vi "运维调试_总磷总氮.vi"() -> ()   [LabVIEW 2016, in "斯坦道通用流路CODmn.lvlib"]
uses:
  <vilib>/Utility/miscctls.llb/LVPointTypeDef.ctl
  <vilib>/Plasmionique/MB Master/MB_Master/MB_Master.lvclass
  <vilib>/ptbypt/NI_PtbyPt.lvlib
panel:
  out "步骤":u16
  out "seconds since 1Jan1904 2":timestamp
  out "seconds since 1Jan1904":timestamp
  in  "周期设置":bool
  in  "流程操作":bool
  out "消解压力":sgl format="%#.2f kPa"
  out "权限等级":string
  out "总步数":i32
  out "滑动杆":dbl(slide) caption="测试进度" scale=0.0..100.0
  out "试剂余量显示":sgl[][](graph)
  in  "仪器校准":bool
  in  "参数查询":bool
  out "简易步骤名称":string
  in  "温度曲线":bool
  in  "试剂余量":bool
  in  "灯值调整":bool
  out "固件版本号":string
  out "模块版本号":string
  out "注射器温度":sgl format="%#.2f ℃"
  out "消解温度":sgl format="%#.2f ℃"
  out "ADC":sgl
  out "F3":sgl format="%#.6f"
  out "F2":sgl format="%#.6f"
  out "F1":sgl format="%#.6f"
  out "F0":sgl format="%#.6f"
  out "运行状态":T1 {"数据时间:" format="%<%y/%m/%d %H:%M:%S>T"; "仪器时间:" format="%<%y/%m/%d %H:%M:%S>T"}
  in  "单选按钮":T2=enum."总氮"
  in  "布尔":bool
  in  "外设固件":bool
  out "字符串 2":string
  in  "数组":string[](array[string])
  in  "返回":bool
  in  "参数设置":bool
  out "集成报警信息":string
  in  "停止":bool
  in  "手动启动":bool
  in  "调试":bool
  out "多列列表框":i32(listbox)
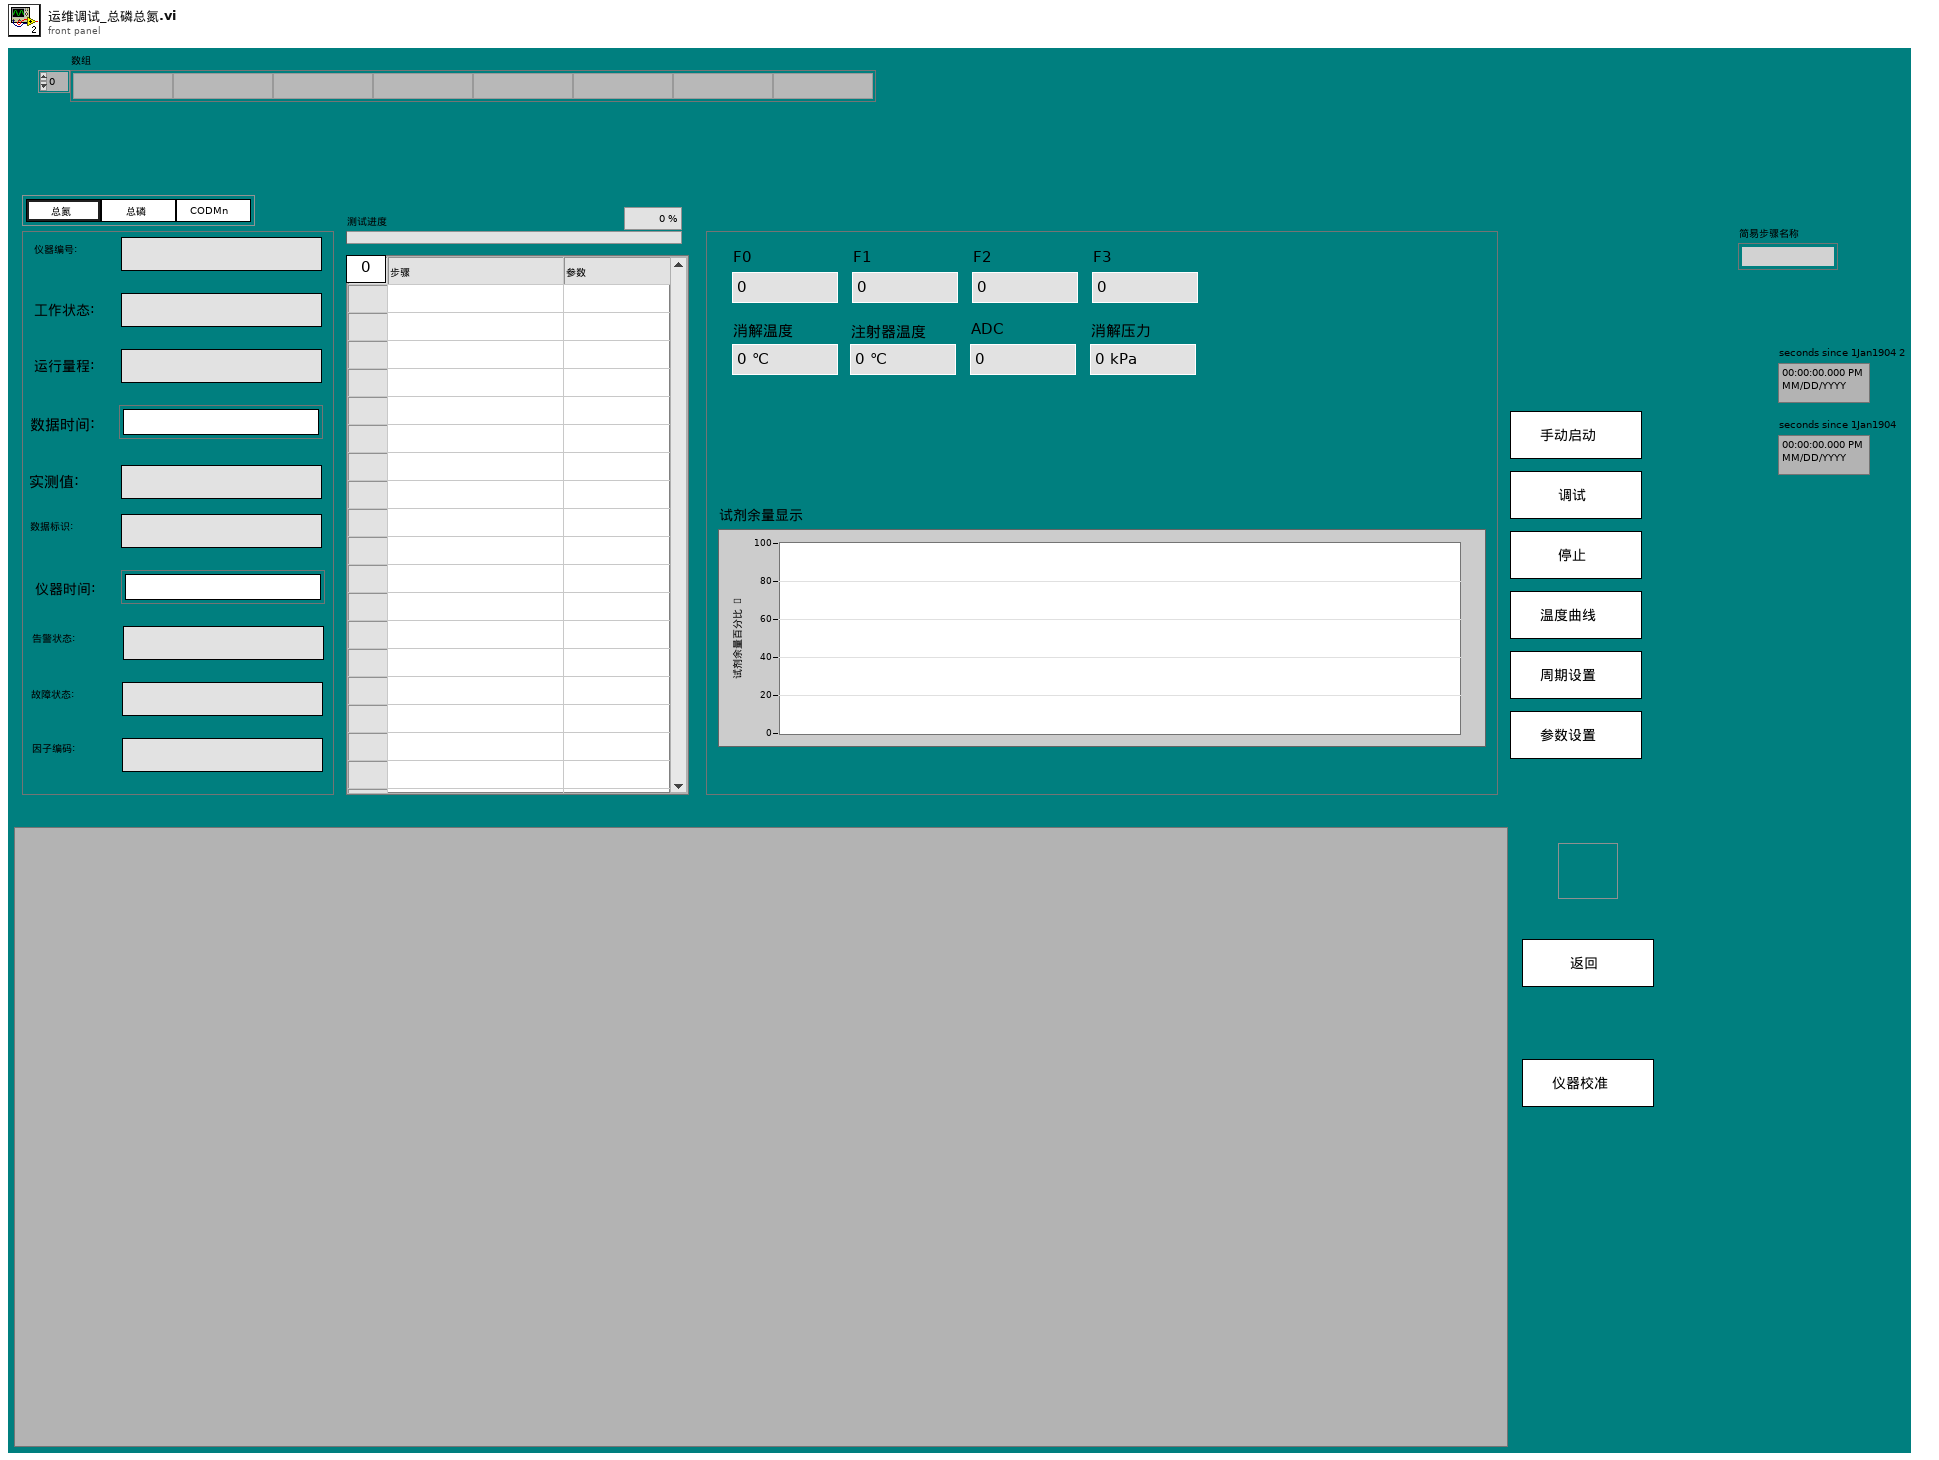
[diagram p1: front panel]
types:
  T1 = cluster{"仪器编号:":string, "工作状态:":string, "运行量程: ":string, "数据时间:":timestamp, "实测值:":string, "数据标识: ":string, "仪器时间:":timestamp, "告警状态: ":string, "故障状态:  ":string, "因子编码:":string}
  T2 = typedef "斯坦道通用流路CODmn.lvlib/启动参数显示控件.ctl" = enum32{"COD", "氨氮", "总氮", "总磷", "磷酸盐", "硝氮", "亚硝氮", "硅酸盐", "硫化物", "氟化物", "CODMn"}
  T3 = cluster{"Major":u16, "Minor":u16, "Fix":u16, "Build":u16}
  T4 = typedef "斯坦道总磷总氮.lvlib/启动参数显示控件.ctl" = enum32{"COD", "氨氮", "总氮", "总磷", "磷酸盐", "硝氮", "亚硝氮", "硅酸盐", "硫化物", "氟化物", "CODMn"}
  T5 = cluster{"系统时间":timestamp, "工作状态":u16, "测量模式":enum16{"待机", "连续模式", "周期模式", "定点模式", "受控模式", "手动模式"}, "告警代码":u16, "故障代码":u16, "日志代码":u16, "软件版本":u16, "F0":sgl, "F1":sgl, "F2":sgl, "F3":sgl, "T":sgl, "H":sgl, "id":u16, "flowid":u16, "量程":u16, "总磷控温温度1":sgl, "营养盐控温温度2":sgl, "ADC":sgl, "结果值":sgl, "运行时间":u16, "步骤详情":string, "步骤流程":string}
  T6 = typedef "LVStringsAndValuesArrayTypeDef_U16.ctl" = cluster{"String":string, "Value":u16}[]
  T7 = typedef "LVPointTypeDef.ctl" = cluster{"Horizontal":i16, "Vertical":i16}
  T8 = cluster{"因子编码":u32, "单位":u16, "标样参考值":sgl, "水样数据时间":timestamp, "水样实测值":sgl, "水样数据标识":string, "标样数据时间":timestamp, "标样实测值":sgl, "标样数据标识":string, "空白数据时间":timestamp, "空白实测值":sgl, "空白数据标识":string, "零点核查数据时间":timestamp, "零点核查实测值":sgl, "零点核查数据标识":string, "跨度核查数据时间":timestamp, "跨度核查实测值":sgl, "跨度核查数据标识":string, "加标回收数据时间":timestamp, "加标回收实测值":sgl, "加标回收数据标识":string, "平行样数据时间":timestamp, "平行样实测值":sgl, "平行样数据标识":string, "F0":sgl, "F1":sgl, "F2":sgl, "F3":sgl, "F4":sgl, "F5":sgl, "F6":sgl, "F7":sgl, "温度":sgl, "湿度":sgl, "X值":sgl, "fidrange":u16, "X1值":sgl}[]
  T9 = typedef "SingleStepTestV3.lvlib/SingleStepTestV3.lvclass/仪器版本.ctl" = enum16{"V3.1版", "V4版", "V3版", "V4.2版"}
  T10 = cluster{"因子编码":u32, "单位":u16, "标样参考值":sgl, "水样数据时间":timestamp, "水样实测值":sgl, "水样数据标识":string, "标样数据时间":timestamp, "标样实测值":sgl, "标样数据标识":string, "空白数据时间":timestamp, "空白实测值":sgl, "空白数据标识":string, "零点核查数据时间":timestamp, "零点核查实测值":sgl, "零点核查数据标识":string, "跨度核查数据时间":timestamp, "跨度核查实测值":sgl, "跨度核查数据标识":string, "加标回收数据时间":timestamp, "加标回收实测值":sgl, "加标回收数据标识":string, "平行样数据时间":timestamp, "平行样实测值":sgl, "平行样数据标识":string, "F0":sgl, "F1":sgl, "F2":sgl, "F3":sgl, "F4":sgl, "F5":sgl, "F6":sgl, "F7":sgl, "温度":sgl, "湿度":sgl, "X值":sgl, "fidrange":u16, "X1值":sgl}
  T11 = typedef "Alarm interface.lvlib/报警短信语音交互.ctl" = cluster{"参数":string, "元器件":string, "故障现象":string, "code":string, "platform_alarm_code":string, "solutionList":cluster{"reason":string, "solution":string}[]}
  T12 = typedef "TimingControl.lvlib/TimingControl.lvclass/国标控制命令.ctl" = enum16{"启动测量", "标样核查", "零点核查", "跨度核查", "空白测试", "平行样测试", "加标回收", "空白校准", "标样校准", "初始化（清洗）", "停止测试", "仪器重启", "校时", "模式设置", "测量间隔设置"}
  T13 = typedef "TimingControl.lvlib/TimingControl.lvclass/测量参数.ctl" = u16
  T14 = enum32{"Bad", "Idle", "Run top level", "Running"}
  T15 = cluster{"时间标识":timestamp, "设备":string, "日志信息":string, "流程参数":string}
  T16 = typedef "LVRowAndColumnUnsignedTypeDef.ctl" = cluster{"Row":u32, "Column":u32}
  T17 = typedef "操作日志字段定义.ctl" = cluster{"时间":timestamp, "参数":string, "日志信息":string, "流程参数":string}
  T18 = cluster{"站号":u16, "量程切换":enum32{"H", "L", "AUTO"}, "控制命令":enum16{"启动测量", "标样核查", "零点核查", "跨度核查", "空白测试", "平行样测试", "加标回收", "空白校准", "标样校准", "初始化（清洗）", "停止测试", "仪器重启", "校时", "模式设置", "测量间隔设置"}, "模式设置":enum16{"待机", "连续模式", "周期模式", "定点模式", "受控模式", "手动模式"}, "测量间隔":u16}
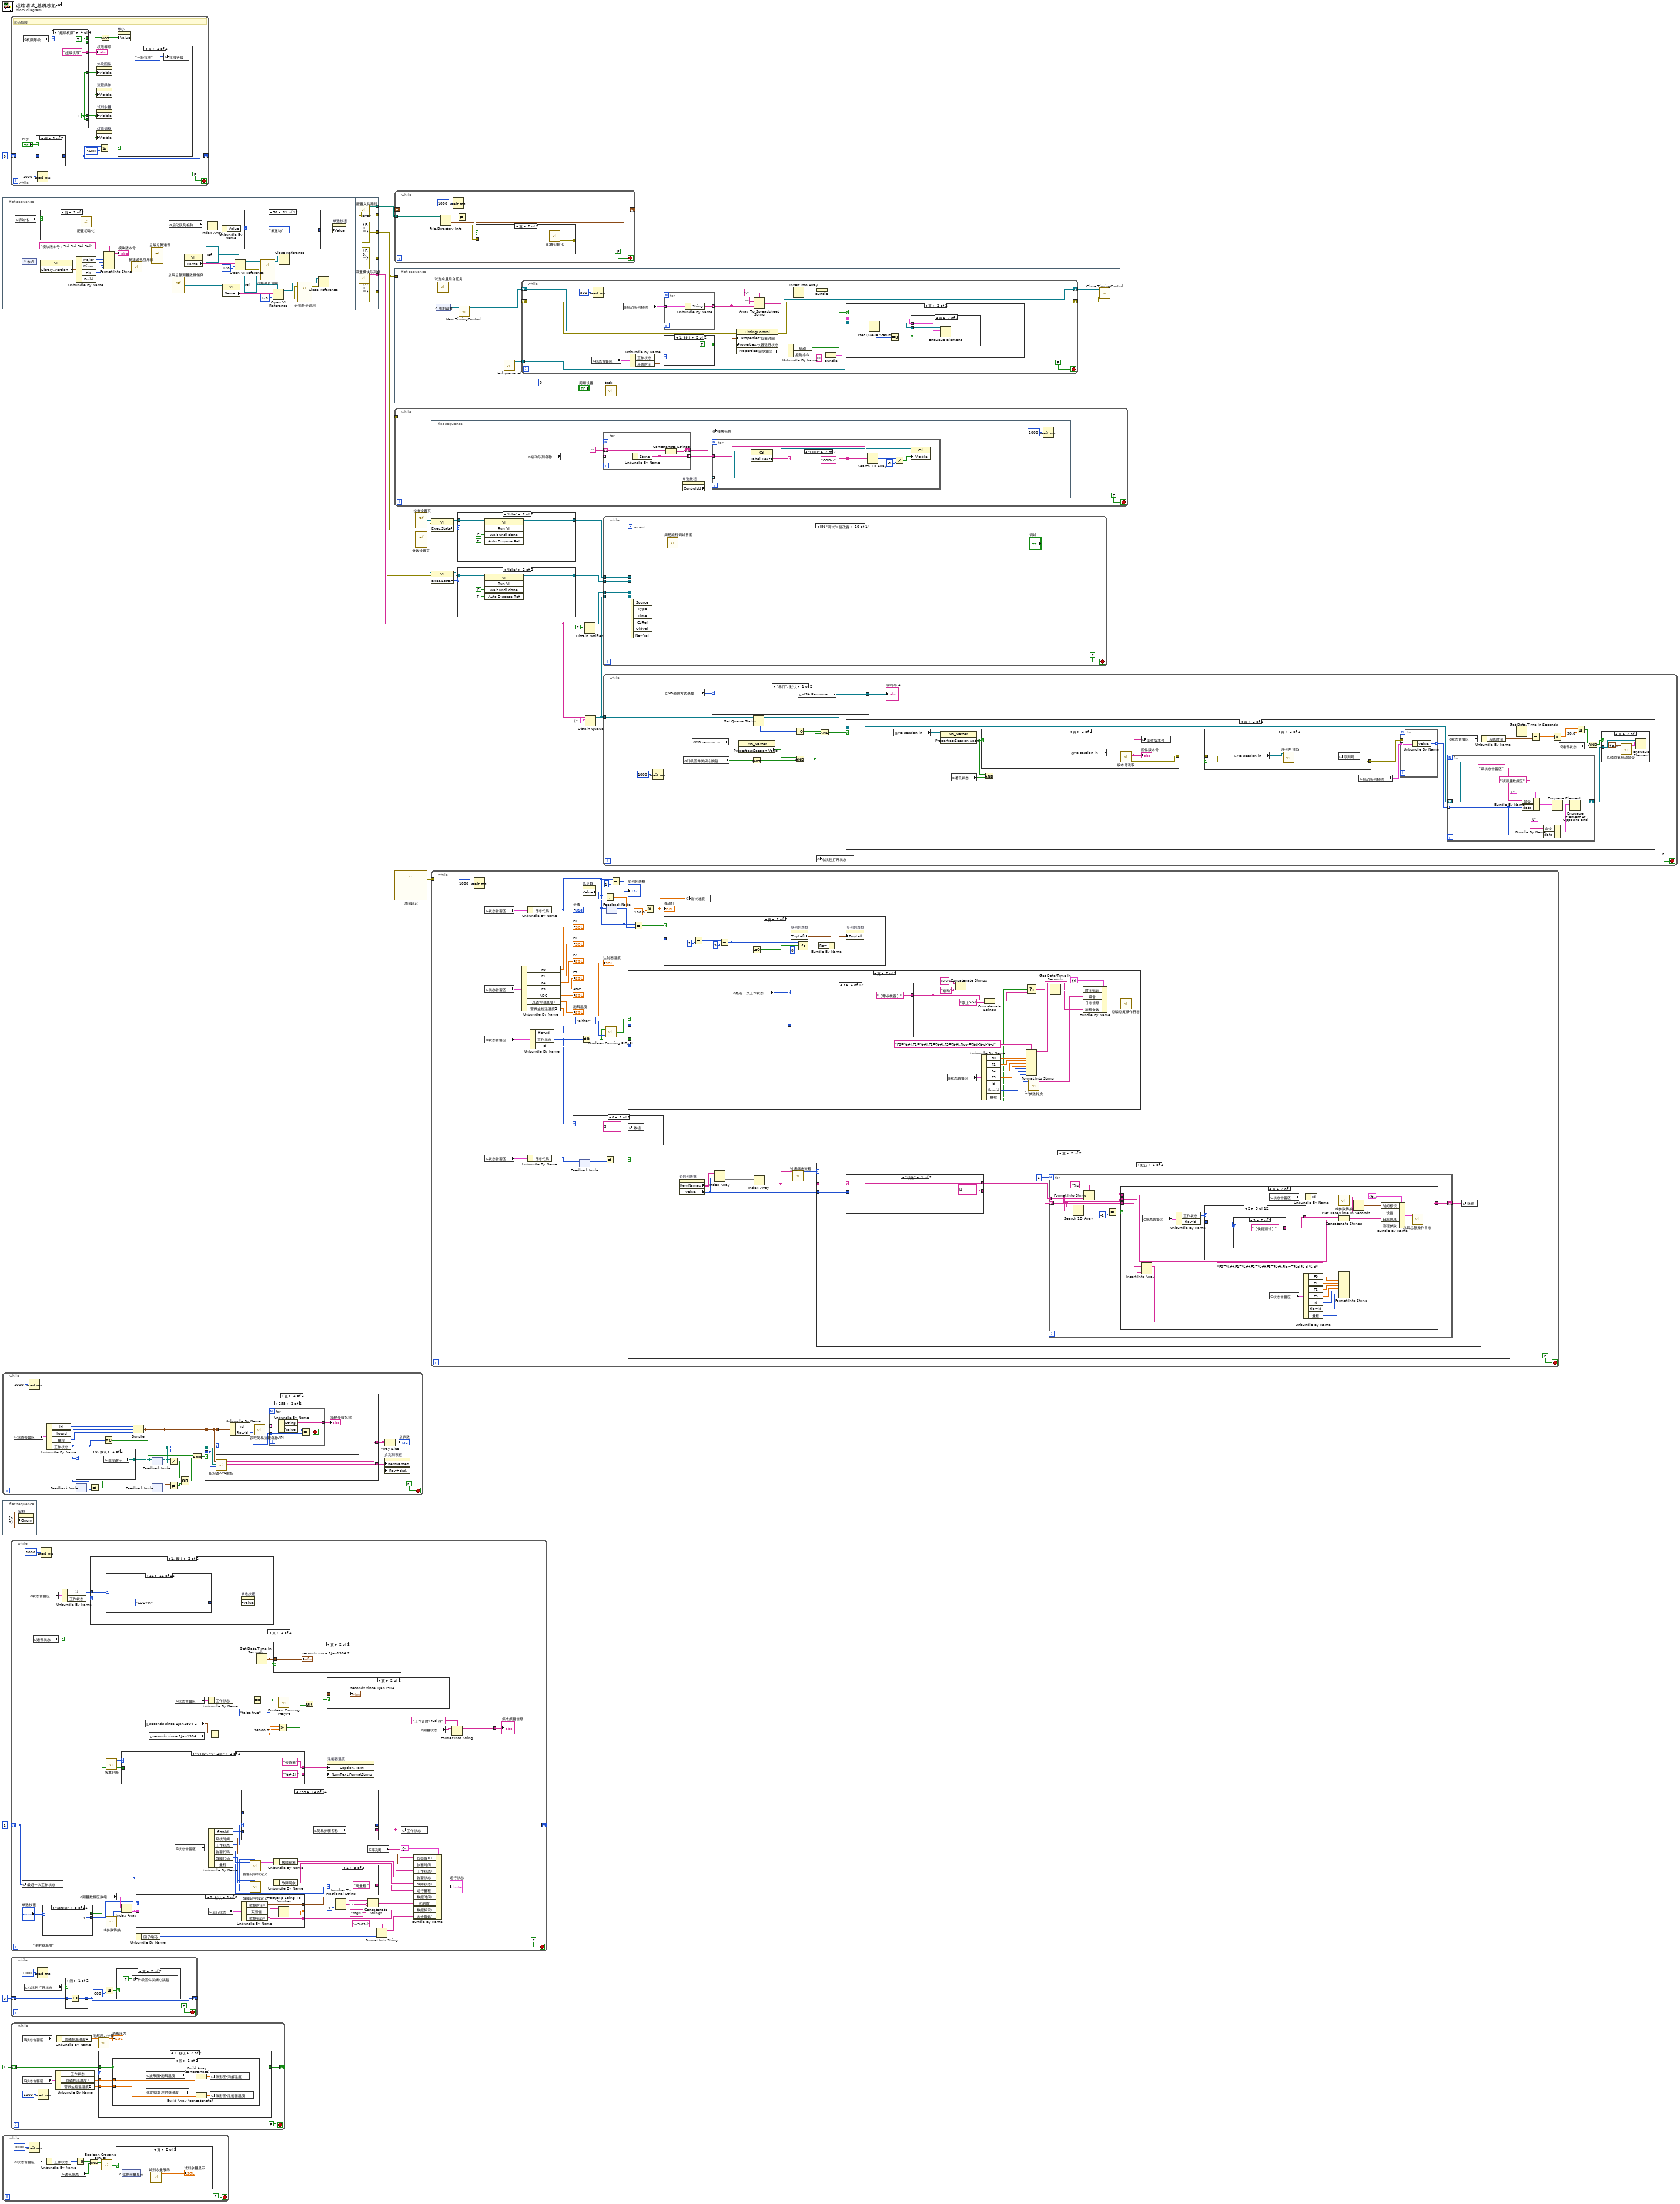
[diagram p0: block diagram]
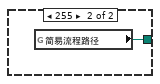
[diagram p2: hidden frame]
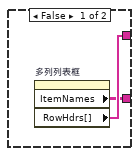
[diagram p3: hidden frame]
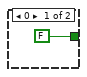
[diagram p7: hidden frame]
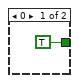
[diagram p14: hidden frame]
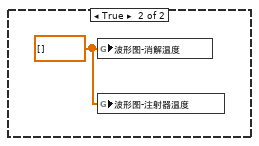
[diagram p15: hidden frame]
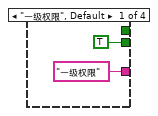
[diagram p17: hidden frame]
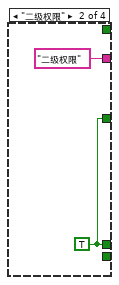
[diagram p18: hidden frame]
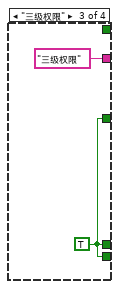
[diagram p19: hidden frame]
diagram:
  n1 = flat-sequence {
    tunnel: [w70] -> w17
    tunnel: [errorcluster {"status"=FALSE, "code"=0, "source"=""} ("错误输入（无错误）")] -> w8
    tunnel: [errorcluster {"status"=FALSE, "code"=0, "source"=""} ("错误输入（无错误）")] -> w7
    tunnel: [w67] -> w5
    tunnel: [errorcluster {"status"=FALSE, "code"=0, "source"=""} ("error out")] -> w4
    tunnel: [errorcluster {"status"=FALSE, "code"=0, "source"=""} ("错误输入（无错误）")] -> w3
    frame #0 {
      n2 = global read "VAR总磷总氮全局变量.vi" "初始化"() -> (w24:bool)
      n3 = control-ref of="本VI"() -> (w32:refnum<vi>)
      n4 = case shown="假" w24 {
        frame False {
          n5 = call "配置初始化.vi"() -> ()  [unwired: 11 in, 1 out]
        }
        frame True {
        }
      }
      n6 = property class="VI"(reference=w32) -> ("Library.Version"=w31:T3)  [unwired: 1 in, 2 out]
      n7 = Unbundle By Name(w31) -> ("Major"=w29:u16, "Minor"=w28:u16, "Fix"=w27:u16, "Build"=w26:u16)
      n8 = Format Into String(format string="模块版本号：%d.%d.%d.%d" ("格式字符串"), w29, w28, w27, w26) -> (resulting string=→"模块版本号":string)  [unwired: 2 in, 1 out]
      n9 = call "新建通讯互斥锁.vi"() -> ()  [unwired: 11 in, 1 out]
    }
    frame #1 {
      n10 = vi-ref "总磷总氮通讯.vi"() -> (w37:refnum<vi>)
      n11 = global read "model config var.vi" "启动队列名称"() -> (w35:cluster{"String":string, "Value":u16}[])
      n12 = vi-ref "总磷总氮测量数据储存.vi"() -> (w45:refnum<vi>)
      n13 = property class="VI"(reference=w37) -> ("Name"=w38:string)  [unwired: 1 in, 2 out]
      n14 = Index Array(array=w35) -> (element=w34:cluster{"String":string, "Value":u16})  [unwired: 1 in]
      n15 = Unbundle By Name(w34) -> ("Value"=w33:u16)
      n16 = property class="VI"(reference=w45) -> ("Name"=w52:string)  [unwired: 1 in, 2 out]
      n17 = Open VI Reference(type specifier VI Refnum (for type only)=refnum<vi> refnum, vi path=w38, options=128 ("选项")) -> (vi reference=w40:refnum<vi>, error out=w42:errorcluster)  [unwired: 3 in]
      n18 = case shown="50" w33 {
        tunnel: [w53 启动参数显示控件."总磷" ("单选按钮") 启动参数显示控件."总氮" ("单选按钮") 启动参数显示控件."COD" ("单选按钮") 启动参数显示控件."氨氮" ("单选按钮") 启动参数显示控件."磷酸盐" ("单选按钮") 启动参数显示控件."硝氮" ("单选按钮") 启动参数显示控件."亚硝氮" ("单选按钮") 启动参数显示控件."硅酸盐" ("单选按钮") 启动参数显示控件."硫化物" ("单选按钮") 启动参数显示控件."氟化物" ("单选按钮") 启动参数显示控件."CODMn" ("单选按钮")] -> w36
        frame 0, Default {
          n19 = property on="单选按钮" class="RadioBtnsControl (严格)"() -> ("Value"=w53:T4)  [unwired: 2 in, 2 out]
        }
        frame 1 {
        }
        frame 2 {
        }
        frame 22 {
        }
        frame 3 {
        }
        frame 4 {
        }
        frame 5 {
        }
        frame 6 {
        }
        frame 7 {
        }
        frame 8 {
        }
        frame 50 {
        }
        frame 21 {
        }
      }
      n20 = call-by-ref "开始异步调用"(reference=w40, error in=w42) -> (reference out=w44:refnum<vi>, error out=w43:errorcluster)  [unwired: 12 in]
      n21 = Open VI Reference(type specifier VI Refnum (for type only)=refnum<vi> refnum, vi path=w52, options=128 ("选项")) -> (vi reference=w50:refnum<vi>, error out=w48:errorcluster)  [unwired: 3 in]
      n22 = Close Reference(reference=w44, error in (no error)=w43) -> ()  [unwired: 1 out]
      n23 = call-by-ref "开始异步调用"(reference=w50, error in=w48) -> (reference out=w46:refnum<vi>, error out=w47:errorcluster)  [unwired: 12 in]
      n24 = Close Reference(reference=w46, error in (no error)=w47) -> ()  [unwired: 1 out]
      n25 = property on="单选按钮" class="RadioBtnsControl (严格)"("Value"=w36) -> ()  [unwired: 2 in, 2 out]
    }
    frame #2 {
      n26 = call "配置文件路径.vi"() -> ("appended path"=w67:path)  [unwired: 11 in]
      n27 = call "设置模块队列名.vi"() -> ("Msg"=w70:string)  [unwired: 5 in]
    }
  }
  n28 = while {
    stop <- FALSE stop-if-true
    n29 = global read "VAR总磷总氮全局变量.vi" "状态告警区"() -> (w82:T5)
    n30 = Wait (ms)(milliseconds to wait=u32 1000 ("等待时间（毫秒）")) -> ()  [unwired: 1 out]
    n31 = Unbundle By Name(w82) -> ("id"=w81:u16, "flowid"=w80:u16, "量程"=w79:u16, "工作状态"=w72:u16)
    n32 = case shown="0, 默认" w72 {
      tunnel: [w92 w93] -> w74
      frame 0, Default {
        n33 = global read "总磷总氮断电保存全局变量.vi" "流程路径"() -> (w92:path)
      }
      frame 255 {
        n34 = global read "总磷总氮断电保存全局变量.vi" "简易流程路径"() -> (w93:path)
      }
    }
    n35 = feedback #1() -> (w71:u16)  [unwired: 1 in]
    n36 = feedback-in #1(w72) -> ()
    n37 = Not Equal?(x=w71, y=w72) -> (x != y?=w88:bool)
    n38 = Not Equal To 0?(x=w72) -> (x != 0?=w83:bool)
    n39 = Bundle("id"=w81, "flowid"=w80, "量程"=w79) -> (w76:cluster{"id":u16, "flowid":u16, "量程":u16})  [unwired: 1 in]
    n40 = feedback #2() -> (w73:path)  [unwired: 1 in]
    n41 = feedback-in #2(w74) -> ()
    n42 = feedback-in #3(w76) -> ()
    n43 = feedback #3() -> (w77:cluster{"id":u16, "flowid":u16, "量程":u16})  [unwired: 1 in]
    n44 = Not Equal?(x=w73, y=w74) -> (x != y?=w87:bool)
    n45 = Not Equal?(x=w76, y=w77) -> (x != y?=w75:bool)
    n46 = Compound Arithmetic op=OR ("复合运算")(w87, w88, w75) -> (w89:bool)
    n47 = And(x=w83, y=w89) -> (x .and. y?=w84:bool)
    n48 = case shown="真" w84 {
      tunnel: [w95 w98] -> w86
      tunnel: [w94 w99] -> w90
      tunnel: w76 -> [_ w97]
      tunnel: w74 -> [_ w100]
      tunnel: w72 -> [_ w96]
      frame False {
        n49 = property on="多列列表框" class="MCListbox (严格)"() -> ("ItemNames"=w94:string[][], "RowHdrs[]"=w95:string[])  [unwired: 2 in, 2 out]
      }
      frame True {
        n50 = case shown="255" w96 {
          tunnel: w97 -> [_ w105]
          frame 0, Default {
          }
          frame 255 {
            n51 = Unbundle By Name(w105) -> ("id"=w104:u16, "flowid"=w102:u16)
            n52 = call "获取简易流程名称API.vi"("参数下拉列表"=w104) -> ("字符串与值[]"=w103:T6)  [unwired: 9 in, 1 out]
            n53 = for {
              tunnel: w103 -> [w110] mode=indexing
              tunnel: w102 -> [w108]
              tunnel: [w107] -> w101
              stop <- w106 stop-if-true
              n54 = Unbundle By Name(w110) -> ("String"=w107:string, "Value"=w109:u16)
              n55 = Equal?(x=w109, y=w108) -> (x = y?=w106:bool)
            }
            "简易步骤名称" <- w101
          }
        }
        n56 = call "斯坦道XML解析.vi"("工作状态"=w96, "添加的路径"=w100, "参数簇"=w97) -> ("步骤名"=w99:string[][], "索引"=w98:string[])  [unwired: 6 in, 1 out]
      }
    }
    n57 = Array Size(array=w86) -> (size(s)=→"总步数":i32)
    n58 = property on="多列列表框" class="MCListbox (严格)"("ItemNames"=w90, "RowHdrs[]"=w86) -> ()  [unwired: 2 in, 2 out]
  }
  n59 = flat-sequence {
    frame #0 {
      n60 = property on="窗格" class="Pane"("Origin"=T7 {"Horizontal"=0, "Vertical"=0} ("原点")) -> ()  [unwired: 2 in, 2 out]
    }
  }
  n61 = while {
    stop <- FALSE stop-if-true
    n62 = global read "VAR总磷总氮全局变量.vi" "状态告警区"() -> (w116:T5)
    n63 = Wait (ms)(milliseconds to wait=u32 1000 ("等待时间（毫秒）")) -> ()  [unwired: 1 out]
    n64 = Unbundle By Name(w116) -> ("工作状态"=w114:u16)
    n65 = global read "VAR总磷总氮全局变量.vi" "通讯状态"() -> (w117:bool)
    n66 = Equal To 0?(x=w114) -> (x = 0?=w113:bool)
    n67 = And(x=w113, y=w117) -> (x .and. y?=w115:bool)
    n68 = call <vilib>:"Boolean Crossing PtByPt.vi"("input"=w115) -> ("crossing"=w112:bool)  [unwired: 2 in]
    n69 = case shown="真" w112 {
      frame False {
      }
      frame True {
        n70 = control-ref of="试剂余量显示"() -> (w120:refnum<vi>)
        n71 = call "试剂余量展示.vi"("波形图 2"=w120) -> ("波形图"=→"试剂余量显示":sgl[][])  [unwired: 10 in]
      }
    }
  }
  n72 = while {
    shift-right: [w131] -> _
    shift-left: u32 0 ("y") -> [w133]
    stop <- FALSE stop-if-true
    # "密码权限"
    n73 = global read "VAR总磷总氮全局变量.vi" "权限等级"() -> (w128:enum16{"一级权限", "二级权限", "三级权限", "超级权限"})
    n74 = case shown="假" "布尔" {
      tunnel: w133 -> [_ w146]
      tunnel: [_ w145] -> w131
      frame False {
      }
      frame True {
        n75 = Increment(x=w146) -> (x+1=w145:u32)
      }
    }
    n76 = Wait (ms)(milliseconds to wait=u32 1000 ("等待时间（毫秒）")) -> ()  [unwired: 1 out]
    n77 = case shown="\"超级权限\"" w128 {
      tunnel: [_ w138 w140 w143] -> w122
      tunnel: [_ _ w140 w143] -> _
      tunnel: [_ w138 w140 w143] -> w127
      tunnel: [_ _ _ TRUE] -> _
      tunnel: [TRUE _ _ _] -> w125
      tunnel: ["一级权限" "二级权限" "三级权限" "超级权限"] -> w123
      frame "一级权限", Default {
      }
      frame "二级权限" {
        w138 = TRUE
      }
      frame "三级权限" {
        w140 = TRUE
      }
      frame "超级权限" {
        w143 = TRUE
      }
    }
    "权限等级" <- w123
    n78 = property on="外设固件" class="Bool"("Visible"=w127) -> ()  [unwired: 2 in, 2 out]
    n79 = property on="流程操作" class="Bool"("Visible"=w122) -> ()  [unwired: 2 in, 2 out]
    n80 = property on="试剂余量" class="Bool"("Visible"=w122) -> ()  [unwired: 2 in, 2 out]
    n81 = property on="灯值调整" class="Bool"("Visible"=w122) -> ()  [unwired: 2 in, 2 out]
    n82 = Greater Or Equal?(x=w131, y=u32 3600) -> (x >= y?=w129:bool)
    n83 = Not(x=w125) -> (.not. x?=w124:bool)
    n84 = property on="布尔" class="Bool (严格)"("Value"=w124) -> ()  [unwired: 2 in, 2 out]
    n85 = case shown="真" w129 {
      frame False {
      }
      frame True {
        n86 = global write "VAR总磷总氮全局变量.vi" "权限等级"(enum16{"一级权限", "二级权限", "三级权限", "超级权限"}."一级权限" ("权限等级")) -> ()
      }
    }
  }
  n87 = while {
    shift-right: [w158] -> _
    shift-left: u16 1 ("工作状态") -> [w156]
    stop <- FALSE stop-if-true
    (unwired) "注射器温度"
    n88 = global write "VAR总磷总氮全局变量.vi" "最近一次工作状态"(w156) -> ()
    n89 = global read "VAR总磷总氮全局变量.vi" "状态告警区"() -> (w178:T5)
    n90 = global read "VAR总磷总氮全局变量.vi" "通讯状态"() -> (w189:bool)
    n91 = Wait (ms)(milliseconds to wait=u32 1000 ("等待时间（毫秒）")) -> ()  [unwired: 1 out]
    n92 = case shown="\"磷酸盐\"" "单选按钮" {
      tunnel: [22 3 2 1 4 5 6 7 8 50 21] -> w147
      tunnel: [_ TRUE _ _ _ _ _ _ _ _ _] -> w150
      frame "COD", Default {
      }
      frame "氨氮" {
      }
      frame "总氮" {
      }
      frame "总磷" {
      }
      frame "磷酸盐" {
      }
      frame "硝氮" {
      }
      frame "亚硝氮" {
      }
      frame "硅酸盐" {
      }
      frame "硫化物" {
      }
      frame "氟化物" {
      }
      frame "CODMn" {
      }
    }
    n93 = Unbundle By Name(w178) -> ("id"=w177:u16, "工作状态"=w173:u16)
    n94 = case shown="真" w189 {
      tunnel: ["通讯异常" ("集成报警信息") w308] -> w188
      frame False {
      }
      frame True {
        n95 = local read "seconds since 1Jan1904 2"() -> (w300:timestamp)
        n96 = local read "seconds since 1Jan1904"() -> (w303:timestamp)
        n97 = global read "VAR总磷总氮全局变量.vi" "状态告警区"() -> (w310:T5)
        n98 = Unbundle By Name(w310) -> ("工作状态"=w306:u16)
        n99 = Subtract(x=w300, y=w303) -> (x-y=w299:dbl)
        n100 = Not Equal To 0?(x=w306) -> (x != 0?=w302:bool)
        n101 = Get Date/Time In Seconds() -> (seconds since 1Jan1904=w301:timestamp)
        n102 = case shown="真" w302 {
          tunnel: w301 -> [_ w311]
          frame False {
          }
          frame True {
            "seconds since 1Jan1904 2" <- w311
          }
        }
        n103 = Greater Or Equal?(x=w299, y=36000.0) -> (x >= y?=w296:bool)
        n104 = call <vilib>:"Boolean Crossing PtByPt.vi"("direction"=enum16{"either", "false-true", "true-false"}."false-true", "input"=w302) -> ("crossing"=w304:bool)  [unwired: 1 in]
        n105 = Or(x=w304, y=w296) -> (x .or. y?=w297:bool)
        n106 = case shown="真" w297 {
          tunnel: w301 -> [_ w312]
          frame False {
          }
          frame True {
            "seconds since 1Jan1904" <- w312
          }
        }
        n107 = global read "VAR总磷总氮全局变量.vi" "测量状态"() -> (w307:string)
        n108 = Format Into String(format string="工作计时: %d 秒" ("格式字符串"), initial string=w307, w299) -> (resulting string=w308:string)  [unwired: 1 in, 1 out]
      }
    }
    "集成报警信息" <- w188
    n109 = global read "VAR总磷总氮全局变量.vi" "测量数据区数组"() -> (w162:T8)
    n110 = case shown="1, 默认" w173 {
      tunnel: w177 -> [_ w245]
      frame 0 {
      }
      frame 1, Default {
        n111 = case shown="21" w245 {
          tunnel: [w246 启动参数显示控件."总磷" ("单选按钮") 启动参数显示控件."总氮" ("单选按钮") 启动参数显示控件."COD" ("单选按钮") 启动参数显示控件."氨氮" ("单选按钮") 启动参数显示控件."磷酸盐" ("单选按钮") 启动参数显示控件."硝氮" ("单选按钮") 启动参数显示控件."亚硝氮" ("单选按钮") 启动参数显示控件."硅酸盐" ("单选按钮") 启动参数显示控件."硫化物" ("单选按钮") 启动参数显示控件."CODMn" ("单选按钮") 启动参数显示控件."氟化物" ("单选按钮")] -> w244
          frame 0, Default {
            n112 = property on="单选按钮" class="RadioBtnsControl (严格)"() -> ("Value"=w246:T4)  [unwired: 2 in, 2 out]
          }
          frame 1 {
          }
          frame 2 {
          }
          frame 22 {
          }
          frame 3 {
          }
          frame 4 {
          }
          frame 5 {
          }
          frame 6 {
          }
          frame 7 {
          }
          frame 8 {
          }
          frame 21 {
          }
          frame 50 {
          }
        }
        n113 = property on="单选按钮" class="RadioBtnsControl (严格)"("Value"=w244) -> ()  [unwired: 2 in, 2 out]
      }
    }
    n114 = call "版本判断.vi"() -> ("仪器版本"=w152:T9)  [unwired: 11 in]
    n115 = call "id参数转换.vi"("id"=w147) -> ("数组资源索引"=w159:i32)  [unwired: 9 in, 1 out]
    n116 = case shown="\"V4版\", \"V4.2版\"" w152 {
      tunnel: [w192 "传感器" ("标题.文本")] -> w149
      tunnel: ["%#.2f ℃" ("数值文本.格式字符串") "%#.2f " ("数值文本.格式字符串")] -> w151
      tunnel: w150 -> [w195 _]
      frame "V3.1版", Default {
        n117 = Select(t="显色温度", s=w195, f="注射器温度" ("标题.文本")) -> (s? t:f=w192:string)
      }
      frame "V4版", "V4.2版" {
      }
    }
    n118 = Index Array(array=w162, index=w159) -> (element=w161:T10)
    n119 = case shown="0, 默认" w156 {
      tunnel: [w213 w219 w223 w227 w231 w235 w239 w243] -> w172
      tunnel: [w211 w218 w222 w226 w229 w234 w238 w242] -> w167
      tunnel: [w214 w217 w221 w225 w228 w233 w237 w241] -> w165
      tunnel: w161 -> [_ w216 w220 w224 w230 w232 w236 w240]
      frame 0, Default {
        n120 = local read "运行状态"() -> (w215:T1)
        n121 = Unbundle By Name(w215) -> ("数据时间:"=w213:timestamp, "实测值:"=w212:string, "数据标识:"=w214:string)
        n122 = Fract/Exp String To Number(string=w212) -> (number=w211:dbl)  [unwired: 3 in, 1 out]
      }
      frame 1 {
        n123 = Unbundle By Name(w216) -> ("水样数据时间"=w219:timestamp, "水样实测值"=w218:sgl, "水样数据标识"=w217:string)
      }
      frame 2, 9 {
        n124 = Unbundle By Name(w220) -> ("标样数据时间"=w223:timestamp, "标样实测值"=w222:sgl, "标样数据标识"=w221:string)
      }
      frame 3 {
        n125 = Unbundle By Name(w224) -> ("零点核查数据时间"=w227:timestamp, "零点核查实测值"=w226:sgl, "零点核查数据标识"=w225:string)
      }
      frame 4 {
        n126 = Unbundle By Name(w230) -> ("跨度核查数据时间"=w231:timestamp, "跨度核查实测值"=w229:sgl, "跨度核查数据标识"=w228:string)
      }
      frame 7 {
        n127 = Unbundle By Name(w232) -> ("加标回收数据时间"=w235:timestamp, "加标回收实测值"=w234:sgl, "加标回收数据标识"=w233:string)
      }
      frame 5, 8 {
        n128 = Unbundle By Name(w236) -> ("空白数据时间"=w239:timestamp, "空白实测值"=w238:sgl, "空白数据标识"=w237:string)
      }
      frame 6 {
        n129 = Unbundle By Name(w240) -> ("平行样数据时间"=w243:timestamp, "平行样实测值"=w242:sgl, "平行样数据标识"=w241:string)
      }
    }
    n130 = Unbundle By Name(w161) -> ("因子编码"=w163:u32)
    n131 = global read "VAR总磷总氮全局变量.vi" "状态告警区"() -> (w187:T5)
    n132 = Unbundle By Name(w187) -> ("flowid"=w155:u16, "系统时间"=w183:timestamp, "工作状态"=w182:u16, "告警代码"=w176:u16, "故障代码"=w175:u16, "量程"=w181:u16)
    n133 = case shown="255" w182 {
      selector: w182 -> [w262 _ w268 w272 w275 w277 w279 w281 w283 w285 w287 w289 w291 w294]
      tunnel: [w263 "空闲" ("工作状态") "水样测量" ("工作状态") w271 "零点核查" ("工作状态") "跨度核查" ("工作状态") "空白测试" ("工作状态") "平行样测试" ("工作状态") "加标回收" ("工作状态") "空白校准" ("工作状态") "标样校准" ("工作状态") "初始化" ("工作状态") "单步调试" ("工作状态") w293] -> w157
      tunnel: [w261 w266 w268 w272 w275 w277 w279 w281 w283 w285 w287 w289 w291 w294] -> w158
      tunnel: w156 -> [w261 w266 _ _ _ _ _ _ _ _ _ _ _ _]
      tunnel: w155 -> [_ _ _ w270 _ _ _ _ _ _ _ _ _ _]
      frame Default {
        n134 = Format Into String(format string="%d" ("格式字符串"), initial string="未知" ("工作状态"), w262) -> (resulting string=w263:string)  [unwired: 1 in, 1 out]
      }
      frame 0 {
      }
      frame 1 {
      }
      frame 2 {
        n135 = case shown="5" w270 {
          tunnel: ["标样核查" ("工作状态") "快捷测试" ("工作状态")] -> w271
          frame 0, Default {
          }
          frame 5 {
          }
        }
      }
      frame 3 {
      }
      frame 4 {
      }
      frame 5 {
      }
      frame 6 {
      }
      frame 7 {
      }
      frame 8 {
      }
      frame 9 {
      }
      frame 10 {
      }
      frame 254 {
      }
      frame 255 {
        n136 = local read "简易步骤名称"() -> (w293:string)
      }
    }
    n137 = call "告警码字段定义.vi"("id"=w147, "告警代码"=w176) -> ("告警信息"=w154:T11)  [unwired: 9 in]
    n138 = call "故障码字段定义.vi"("id"=w147, "故障代码"=w175) -> ("告警信息"=w174:T11)  [unwired: 9 in]
    n139 = Unbundle By Name(w154) -> ("故障现象"=w153:string)
    n140 = Unbundle By Name(w174) -> ("故障现象"=w148:string)
    n141 = property on="注射器温度" class="DigNum (严格)"("Caption.Text"=w149, "NumText.FormatString"=w151) -> ()  [unwired: 2 in, 2 out]
    n142 = case shown="1" w181 {
      tunnel: ["" ("字符串") "低量程 " ("字符串") "高量程 " ("字符串")] -> w180
      frame Default {
      }
      frame 0 {
      }
      frame 1 {
      }
    }
    n143 = Number To Fractional String(number=w167, precision (6)=i16 4 ("精度(6)")) -> (F-format string=w169:string)  [unwired: 2 in]
    n144 = Concatenate Strings(w169, " " ("字符串"), "mg/L" ("字符串")) -> (w166:string)
    n145 = global read "VAR总磷总氮全局变量.vi" "序列号"() -> (w184:string)
    n146 = Format Into String(format string="w%05d" ("格式字符串"), w163) -> (resulting string=w179:string)  [unwired: 2 in, 1 out]
    n147 = global write "VAR总磷总氮全局变量.vi" "工作状态:"(w157) -> ()
    n148 = Bundle By Name(cluster=T1 {"仪器编号:"="", "工作状态:"="", "运行量程: "="", "数据时间:"=timestamp(0 s since 1904-01-01), "实测值:"="", "数据标识: "="", "仪器时间:"=timestamp(0 s since 1904-01-01), "告警状态: "="", "故障状态:  "="", "因子编码:"=""} ("运行状态"), "仪器编号:"=w184, "仪器时间:"=w183, "工作状态:"=w157, "告警状态:"=w153, "故障状态:"=w148, "运行量程:"=w180, "数据时间:"=w172, "实测值:"=w166, "数据标识:"=w165, "因子编码:"=w179) -> (→"运行状态":T1)
  }
  n149 = while {
    shift-right: [w317] -> _
    shift-left: 0 -> [w318]
    stop <- FALSE stop-if-true
    n150 = global read "VAR总磷总氮全局变量.vi" "心跳包打开状态"() -> (w313:bool)
    n151 = Wait (ms)(milliseconds to wait=u32 1000 ("等待时间（毫秒）")) -> ()  [unwired: 1 out]
    n152 = case shown="假" w313 {
      tunnel: w318 -> [w322 _]
      tunnel: [w321 _] -> w317
      frame False {
        n153 = Increment(x=w322) -> (x+1=w321:i32)
      }
      frame True {
      }
    }
    n154 = Greater Or Equal?(x=w317, y=600) -> (x >= y?=w315:bool)
    n155 = case shown="真" w315 {
      frame False {
      }
      frame True {
        n156 = global write "VAR总磷总氮全局变量.vi" "升级固件关闭心跳包"(FALSE ("关闭心跳包")) -> ()
      }
    }
  }
  n157 = while {
    shift-right: [w324] -> _
    shift-left: TRUE -> [w325]
    stop <- FALSE stop-if-true
    n158 = global read "VAR总磷总氮全局变量.vi" "状态告警区"() -> (w328:T5)
    n159 = global read "VAR总磷总氮全局变量.vi" "状态告警区"() -> (w331:T5)
    n160 = Wait (ms)(milliseconds to wait=u32 1000 ("等待时间（毫秒）")) -> ()  [unwired: 1 out]
    n161 = Unbundle By Name(w331) -> ("工作状态"=w326:u16, "总磷控温温度1"=w330:sgl, "营养盐控温温度2"=w329:sgl)
    n162 = Unbundle By Name(w328) -> ("总磷控温温度1"=w327:sgl)
    n163 = call "消解压力计算.vi"("当前消解温度"=w327) -> ("消解压力"=→"消解压力":dbl)  [unwired: 10 in]
    n164 = case shown="1, 默认" w326 {
      tunnel: w330 -> [_ w337]
      tunnel: w329 -> [_ w336]
      tunnel: w325 -> [_ w335]
      tunnel: [TRUE _] -> w324
      frame 0 {
      }
      frame 1, Default {
        n165 = case shown="假" w335 {
          tunnel: w337 -> [w343 _]
          tunnel: w336 -> [w342 _]
          frame False {
            n166 = global read "VAR总磷总氮全局变量.vi" "波形图-消解温度"() -> (w341:sgl[])
            n167 = global read "VAR总磷总氮全局变量.vi" "波形图-注射器温度"() -> (w340:sgl[])
            n168 = Build Array (concatenate)(w341, w343) -> (w339:sgl[])
            n169 = Build Array (concatenate)(w340, w342) -> (w338:sgl[])
            n170 = global write "VAR总磷总氮全局变量.vi" "波形图-消解温度"(w339) -> ()
            n171 = global write "VAR总磷总氮全局变量.vi" "波形图-注射器温度"(w338) -> ()
          }
          frame True {
            w344 = dbl[] [] ("波形图-消解温度")
            n172 = global write "VAR总磷总氮全局变量.vi" "波形图-消解温度"(w344) -> ()
            n173 = global write "VAR总磷总氮全局变量.vi" "波形图-注射器温度"(w344) -> ()
          }
        }
      }
    }
  }
  n174 = while {
    shift-right: [w345] -> _
    shift-left: _ -> [w350]
    tunnel: w5 -> [w348]
    stop <- FALSE stop-if-true
    n175 = File/Directory Info(path=w348) -> (last mod=w345:timestamp, error out=w346:errorcluster)  [unwired: 1 in, 5 out]
    n176 = Wait (ms)(milliseconds to wait=u32 1000 ("等待时间（毫秒）")) -> ()  [unwired: 1 out]
    n177 = Not Equal?(x=w350, y=w345) -> (x != y?=w349:bool)
    n178 = case shown="真" w349 {
      tunnel: [_ w352] -> _
      tunnel: w346 -> [_ _]
      frame False {
      }
      frame True {
        n179 = call "配置初始化.vi"() -> ("error out"=w352:errorcluster)  [unwired: 11 in]
      }
    }
  }
  n180 = flat-sequence {
    tunnel: w4 -> [_]
    frame #0 {
      (unwired) u32 0 ("等待时间（毫秒）")
      n181 = control-ref of="周期设置"() -> (w357:refnum<vi>)
      n182 = call "试剂余量后台任务.vi"() -> ()  [unwired: 12 in]
      n183 = call "New TimingControl.vi"("Reference"=w357) -> ("error out"=w355:errorcluster, "TimingControl out"=w356:refnum<class "TimingControl.lvclass">)  [unwired: 9 in]
      n184 = call "taskqueue ref.vi"() -> ("队列输出"=w358:refnum<queue>)  [unwired: 10 in, 1 out]
      n185 = while {
        tunnel: w358 -> [w377]
        shift-right: [w370] -> w354
        shift-left: w356 -> [w375]
        shift-right: [w369] -> w353
        shift-left: w355 -> [w374]
        stop <- FALSE stop-if-true
        n186 = global read "VAR总磷总氮全局变量.vi" "状态告警区"() -> (w378:T5)
        n187 = Wait (ms)(milliseconds to wait=u32 500 ("等待时间（毫秒）")) -> ()  [unwired: 1 out]
        n188 = global read "model config var.vi" "启动队列名称"() -> (w364:cluster{"String":string, "Value":u16}[])
        n189 = Unbundle By Name(w378) -> ("工作状态"=w376:u16, "系统时间"=w372:timestamp)
        n190 = for {
          tunnel: w364 -> [w389] mode=indexing
          tunnel: [w388] -> w363 mode=indexing
          n191 = Unbundle By Name(w389) -> ("String"=w388:string)
        }
        n192 = case shown="1, 默认" w376 {
          tunnel: [FALSE TRUE] -> w371
          frame 0 {
          }
          frame 1, Default {
          }
        }
        n193 = property class="TimingControl"(reference=w375, error in=w374, "Properties:仪器时间"=w372, "Properties:仪器运行状态"=w371) -> (reference out=w370:refnum<class "TimingControl.lvclass">, error out=w369:errorcluster, "Properties:命令输出"=w373:cluster{"启动":bool, "控制命令":T12, "测量参数":T13})
        n194 = Array To Spreadsheet String(delimiter (Tab)="/" ("分隔符(Tab)"), array=w363, 3:"" ("格式字符串")) -> (spreadsheet string=w366:string)
        n195 = Unbundle By Name(w373) -> ("启动"=w360:bool, "控制命令"=w362:T12)
        n196 = Insert Into Array(array=w363, new element=w366) -> (w365:string[])  [unwired: 1 in]
        n197 = Bundle(w365) -> ()  [unwired: 1 in, 1 out]
        n198 = Bundle("控制命令"=w362, "") -> (w361:cluster{"控制命令":T12, string})  [unwired: 1 in]
        n199 = case shown="真" w360 {
          tunnel: w361 -> [_ w382]
          tunnel: w377 -> [_ w385]
          frame False {
          }
          frame True {
            n200 = Get Queue Status(queue=w385) -> (queue out=w383:refnum<queue>, # elements in queue=w384:i32)  [unwired: 2 in, 6 out]
            n201 = Equal To 0?(x=w384) -> (x = 0?=w381:bool)
            n202 = case shown="真" w381 {
              tunnel: w383 -> [_ w387]
              tunnel: w382 -> [_ w386]
              frame False {
              }
              frame True {
                n203 = Enqueue Element(queue=w387, element=w386) -> ()  [unwired: 2 in, 3 out]
              }
            }
          }
        }
      }
      n204 = call "task.vi"() -> ()  [unwired: 12 in]
      n205 = call "Close TimingControl.vi"("error in (no error)"=w353, "TimingControl in"=w354) -> ()  [unwired: 9 in, 1 out]
    }
  }
  n206 = while {
    tunnel: w4 -> [_]
    stop <- FALSE stop-if-true
    n207 = flat-sequence {
      frame #0 {
        n208 = global read "model config var.vi" "启动队列名称"() -> (w393:cluster{"String":string, "Value":u16}[])
        n209 = for {
          tunnel: w393 -> [w401] mode=indexing
          shift-right: [w400] -> w396
          shift-left: "" -> [w399]
          tunnel: [w398] -> w394 mode=indexing
          n210 = Unbundle By Name(w401) -> ("String"=w398:string)
          n211 = Concatenate Strings(w399, w398) -> (w400:string)
        }
        n212 = property on="单选按钮" class="RadioBtnsControl (严格)"() -> ("Controls[]"=w395:refnum<vi>[])  [unwired: 2 in, 2 out]
        n213 = global write "VAR总磷总氮全局变量.vi" "模块名称"(w396) -> ()
        n214 = for {
          tunnel: w395 -> [w409] mode=indexing
          tunnel: w394 -> [w408]
          n215 = property class="Ctl"(reference=w409) -> (reference out=w407:refnum<vi>, "Label.Text"=w403:string)  [unwired: 1 in, 1 out]
          n216 = case shown="\"COD\"" w403 {
            selector: w403 -> [w410 _]
            tunnel: [w410 "CODcr"] -> w402
            frame Default {
            }
            frame "COD" {
            }
          }
          n217 = Search 1D Array(1D array=w408, element=w402) -> (index of element=w406:i32)  [unwired: 1 in]
          n218 = Not Equal?(x=w406, y=-1) -> (x != y?=w404:bool)
          n219 = property class="Ctl"(reference=w407, "Visible"=w404) -> ()  [unwired: 1 in, 2 out]
        }
      }
      frame #1 {
        n220 = Wait (ms)(milliseconds to wait=u32 1000 ("等待时间（毫秒）")) -> ()  [unwired: 1 out]
      }
    }
  }
  n221 = call "时间延迟"("error in (no error)"=w3) -> ("error out"=w23:errorcluster)  [unwired: 10 in]
  n222 = vi-ref "校准设置页.vi"() -> (w12:refnum<vi>)
  n223 = vi-ref "参数设置页.vi"() -> (w16:refnum<vi>)
  n224 = property class="VI"(reference=w12, error in=w7) -> (reference out=w10:refnum<vi>, "Exec.State"=w11:T14)  [unwired: 1 out]
  n225 = property class="VI"(reference=w16, error in=w8) -> (reference out=w14:refnum<vi>, "Exec.State"=w15:T14)  [unwired: 1 out]
  n226 = while {
    tunnel: w23 -> [_]
    stop <- FALSE stop-if-true
    n227 = Wait (ms)(milliseconds to wait=u32 1000 ("等待时间（毫秒）")) -> ()  [unwired: 1 out]
    n228 = global read "VAR总磷总氮全局变量.vi" "状态告警区"() -> (w438:T5)
    n229 = global read "VAR总磷总氮全局变量.vi" "状态告警区"() -> (w439:T5)
    n230 = global read "VAR总磷总氮全局变量.vi" "状态告警区"() -> (w437:T5)
    n231 = global read "VAR总磷总氮全局变量.vi" "状态告警区"() -> (w435:T5)
    n232 = Unbundle By Name(w439) -> ("F0"=→"F0":sgl, "F1"=→"F1":sgl, "F2"=→"F2":sgl, "F3"=→"F3":sgl, "ADC"=→"ADC":sgl, "总磷控温温度1"=→"消解温度":sgl, "营养盐控温温度2"=→"注射器温度":sgl)
    n233 = Unbundle By Name(w438) -> ("日志代码"=w413:u16)
    "步骤" <- w413
    n234 = Unbundle By Name(w435) -> ("日志代码"=w434:u16)
    n235 = Unbundle By Name(w437) -> ("flowid"=w417:u16, "工作状态"=w430:u16, "id"=w431:u16)
    n236 = case shown="0" w430 {
      frame 0 {
        n237 = local write "数组"(string[] [] ("数组")) -> ()
      }
      frame 1, Default {
      }
    }
    n238 = feedback #4() -> (w436:u16)  [unwired: 1 in]
    n239 = feedback-in #4(w434) -> ()
    n240 = Not Equal To 0?(x=w430) -> (x != 0?=w415:bool)
    n241 = property on="总步数" class="DigNum (严格)"() -> ("Value"=w420:i32)  [unwired: 2 in, 2 out]
    n242 = Divide(x=w413, y=w420) -> (x/y=w419:dbl)
    n243 = Not Equal?(x=w434, y=w436) -> (x != y?=w433:bool)
    n244 = call <vilib>:"Boolean Crossing PtByPt.vi"("direction"=enum16{"either", "false-true", "true-false"}."either", "input"=w415) -> ("crossing"=w428:bool)  [unwired: 1 in]
    n245 = feedback-in #5(w413) -> ()
    n246 = feedback #5() -> (w441:u16)  [unwired: 1 in]
    n247 = Subtract(x=w413, y=1) -> (x-y=→"多列列表框":i32)
    n248 = case shown="真" w428 {
      tunnel: w431 -> [_ w464]
      tunnel: w417 -> [_ w452]
      tunnel: w415 -> [_ w450]
      frame False {
      }
      frame True {
        n249 = global read "VAR总磷总氮全局变量.vi" "最近一次工作状态"() -> (w451:u16)
        n250 = case shown="3" w451 {
          selector: w451 -> [w470 _ _ _ _ _ _ _ _ _ _ _]
          tunnel: [w469 "【水样测试】" ("字符串") w473 "【零点核查】" ("字符串") "【跨度核查】" ("字符串") "【空白测试】" ("字符串") "【平行样测试】" ("字符串") "【加标回收】" ("字符串") "【空白校准】" ("字符串") "【标样校准】" ("字符串") "【单步调试】" ("字符串") "【简易流程】" ("字符串")] -> w445
          tunnel: w452 -> [_ _ w472 _ _ _ _ _ _ _ _ _]
          frame 0, Default {
            n251 = Number To Decimal String(number=w470) -> (decimal integer string=w469:string)  [unwired: 1 in]
          }
          frame 1 {
          }
          frame 2 {
            n252 = case shown="0, 默认" w472 {
              tunnel: ["【标样核查】" ("字符串") "【快捷测试】" ("字符串")] -> w473
              frame 0, Default {
              }
              frame 5 {
              }
            }
          }
          frame 3 {
          }
          frame 4 {
          }
          frame 5 {
          }
          frame 6 {
          }
          frame 7 {
          }
          frame 8 {
          }
          frame 9 {
          }
          frame 254 {
          }
          frame 255 {
          }
        }
        n253 = global read "VAR总磷总氮全局变量.vi" "状态告警区"() -> (w462:T5)
        n254 = Concatenate Strings("<<" ("字符串"), w445, "启动" ("字符串")) -> (w444:string)
        n255 = Unbundle By Name(w462) -> ("F0"=w461:sgl, "F1"=w460:sgl, "F2"=w459:sgl, "F3"=w458:sgl, "id"=w457:u16, "flowid"=w456:u16, "量程"=w455:u16)
        n256 = Concatenate Strings(w445, "停止>>" ("字符串")) -> (w448:string)
        n257 = Format Into String(format string="F0=%#f,F1=%#f,F2=%#f,F3=%#f,Flow=%d-%-d-%-d" ("格式字符串"), w461, w460, w459, w458, w457, w456, w455) -> (resulting string=w453:string)  [unwired: 2 in, 1 out]
        n258 = Select(t=w444, s=w450, f=w448) -> (s? t:f=w449:string)
        n259 = call "id参数转换.vi"("id"=w464) -> ("table输出"=w463:string)  [unwired: 9 in, 1 out]
        n260 = Get Date/Time In Seconds() -> (seconds since 1Jan1904=w467:timestamp)
        n261 = Bundle By Name(cluster=T15 {"时间标识"=timestamp(0 s since 1904-01-01), "设备"="", "日志信息"="", "流程参数"=""} ("data in"), "时间标识"=w467, "设备"=w463, "日志信息"=w449, "流程参数"=w453) -> (w466:T15)
        n262 = call "总磷总氮操作日志.vi"("data in"=w466) -> ()  [unwired: 10 in, 1 out]
      }
    }
    n263 = case shown="真" w433 {
      frame False {
      }
      frame True {
        n264 = property on="多列列表框" class="MCListbox (严格)"() -> ("ItemNames"=w490:string[][], "Value"=w486:i32)  [unwired: 2 in, 2 out]
        n265 = Index Array(array=w490, index (row)=w486) -> (element=w489:string[])  [unwired: 1 in]
        n266 = Index Array(array=w489) -> (element=w488:string)  [unwired: 1 in]
        n267 = call "过滤筛选流程.vi"("字符串"=w488) -> ("匹配后偏移量"=w487:i32)  [unwired: 10 in]
        n268 = case shown="默认" w487 {
          tunnel: w488 -> [w492 _]
          tunnel: w486 -> [w491 _]
          frame Default {
            n269 = case shown="\"读数\"" w492 {
              selector: w492 -> [w498 w505]
              tunnel: [w498 w505] -> w494
              tunnel: [string[] [] ("数组") w500] -> w493
              tunnel: w491 -> [_ w504]
              frame "读数" {
              }
              frame Default {
                n270 = Equal?(x=w504, y=1) -> (x = y?=w502:bool)
                n271 = Select(t=string[] [], s=w502, f="数组") -> (s? t:f=w500:string[])
              }
            }
            n272 = for {
              N: 1 -> [_]
              tunnel: w494 -> [w507]
              shift-right: [w506] -> w495
              shift-left: w493 -> [w508]
              n273 = Search 1D Array(1D array=w508, element=w507) -> (index of element=w511:i32)  [unwired: 1 in]
              n274 = Format Into String(format string="%s" ("格式字符串"), w507) -> (resulting string=w512:string)  [unwired: 2 in, 1 out]
              n275 = Equal?(x=w511, y=-1) -> (x = y?=w509:bool)
              n276 = case shown="真" w509 {
                tunnel: w512 -> [_ w522]
                tunnel: w508 -> [w514 w526]
                tunnel: w507 -> [_ w525]
                tunnel: [w514 w524] -> w506
                frame False {
                }
                frame True {
                  n277 = Insert Into Array(array=w526, new element=w525) -> (w524:string[])  [unwired: 1 in]
                  n278 = global read "VAR总磷总氮全局变量.vi" "状态告警区"() -> (w521:T5)
                  n279 = Unbundle By Name(w521) -> ("工作状态"=w520:u16, "flowid"=w515:u16)
                  n280 = case shown="2" w520 {
                    selector: w520 -> [w541 _ _ _ _ _ _ _ _ _ _ _]
                    tunnel: [w540 "【水样测试】" ("字符串") w544 "【零点核查】" ("字符串") "【跨度核查】" ("字符串") "【空白测试】" ("字符串") "【平行样测试】" ("字符串") "【加标回收】" ("字符串") "【空白校准】" ("字符串") "【标样校准】" ("字符串") "【单步调试】" ("字符串") w555] -> w518
                    tunnel: w515 -> [_ _ w543 _ _ _ _ _ _ _ _ _]
                    frame 0, Default {
                      n281 = Number To Decimal String(number=w541) -> (decimal integer string=w540:string)  [unwired: 1 in]
                    }
                    frame 1 {
                    }
                    frame 2 {
                      n282 = case shown="5" w543 {
                        tunnel: ["【标样核查】" ("字符串") "【快捷测试】" ("字符串")] -> w544
                        frame Default {
                        }
                        frame 5 {
                        }
                      }
                    }
                    frame 3 {
                    }
                    frame 4 {
                    }
                    frame 5 {
                    }
                    frame 6 {
                    }
                    frame 7 {
                    }
                    frame 8 {
                    }
                    frame 9 {
                    }
                    frame 254 {
                    }
                    frame 255 {
                      n283 = local read "简易步骤名称"() -> (w557:string)
                      n284 = Format Into String(format string="(%s)" ("格式字符串"), initial string="【简易流程】" ("工作状态"), w557) -> (resulting string=w555:string)  [unwired: 1 in, 1 out]
                    }
                  }
                  n285 = global read "VAR总磷总氮全局变量.vi" "状态告警区"() -> (w539:T5)
                  n286 = global read "VAR总磷总氮全局变量.vi" "状态告警区"() -> (w536:T5)
                  n287 = Unbundle By Name(w536) -> ("F0"=w533:sgl, "F1"=w532:sgl, "F2"=w531:sgl, "F3"=w530:sgl, "id"=w529:u16, "flowid"=w528:u16, "量程"=w527:u16)
                  n288 = Unbundle By Name(w539) -> ("id"=w517:u16)
                  n289 = call "id参数转换.vi"("id"=w517) -> ("table输出"=w516:string)  [unwired: 9 in, 1 out]
                  n290 = Concatenate Strings(w518, w522) -> (w519:string)
                  n291 = Format Into String(format string="F0=%#f,F1=%#f,F2=%#f,F3=%#f,Flow=%d-%-d-%-d" ("格式字符串"), w533, w532, w531, w530, w529, w528, w527) -> (resulting string=w534:string)  [unwired: 2 in, 1 out]
                  n292 = Get Date/Time In Seconds() -> (seconds since 1Jan1904=w537:timestamp)
                  n293 = Bundle By Name(cluster=T15 {"时间标识"=timestamp(0 s since 1904-01-01), "设备"="", "日志信息"="", "流程参数"=""} ("data in"), "时间标识"=w537, "设备"=w516, "日志信息"=w519, "流程参数"=w534) -> (w538:T15)
                  n294 = call "总磷总氮操作日志.vi"("data in"=w538) -> ()  [unwired: 10 in, 1 out]
                }
              }
            }
            n295 = local write "数组"(w495) -> ()
          }
          frame -1 {
          }
        }
      }
    }
    n296 = Not Equal?(x=w413, y=w441) -> (x != y?=w440:bool)
    n297 = Multiply(x=w419, y=100.0) -> (x*y=w416:dbl)
    "滑动杆" <- w416
    n298 = case shown="真" w440 {
      tunnel: w413 -> [_ w561]
      frame False {
      }
      frame True {
        n299 = Subtract(x=w561, y=1) -> (x-y=w559:i32)
        n300 = Subtract(x=w559, y=5) -> (x-y=w563:i32)
        n301 = Greater Or Equal To 0?(x=w563) -> (x >= 0?=w562:bool)
        n302 = property on="多列列表框" class="MCListbox (严格)"() -> (error out=w567:errorcluster, "TopLeft"=w568:T16)  [unwired: 2 in, 1 out]
        n303 = Select(t=w563, s=w562, f=0) -> (s? t:f=w564:i32)
        n304 = Bundle By Name(cluster=w568, "Row"=w564) -> (w569:T16)
        n305 = property on="多列列表框" class="MCListbox (严格)"(error in=w567, "TopLeft"=w569) -> ()  [unwired: 1 in, 2 out]
      }
    }
    n306 = global write "VAR总磷总氮全局变量.vi" "测试进度"(w416) -> ()
  }
  n307 = case shown="\"Idle\"" w11 {
    tunnel: w10 -> [w570 w574]
    tunnel: [w570 w571] -> w9
    frame "Bad", Default {
    }
    frame "Idle" {
      n308 = invoke class="VI" method="Run VI"(reference=w574, "Wait until done"=FALSE ("结束前等待"), "Auto Dispose Ref"=TRUE ("自动销毁引用")) -> (reference out=w571:refnum<vi>)  [unwired: 2 in, 4 out]
    }
  }
  n309 = case shown="\"Idle\"" w15 {
    tunnel: w14 -> [w575 w579]
    tunnel: [w575 w576] -> w13
    frame "Bad", Default {
    }
    frame "Idle" {
      n310 = invoke class="VI" method="Run VI"(reference=w579, "Wait until done"=FALSE ("结束前等待"), "Auto Dispose Ref"=TRUE ("自动销毁引用")) -> (reference out=w576:refnum<vi>)  [unwired: 2 in, 4 out]
    }
  }
  n311 = Obtain Notifier(name (unnamed)=w17, notification data type=FALSE) -> (notifier out=w18:refnum<notifier>)  [unwired: 2 in, 2 out]
  n312 = Obtain Queue(name (unnamed)=w17, element data type=cluster{"命令":string, "data":variant} {"命令"="", "data"=variant}) -> (queue out=w20:refnum<queue>)  [unwired: 3 in, 2 out]
  n313 = while {
    tunnel: w20 -> [w583]
    tunnel: w18 -> [w582]
    tunnel: w13 -> [w581]
    tunnel: w9 -> [w580]
    stop <- FALSE stop-if-true
    n314 = event shown="[9] \"调试\": 值改变" {
      selector: _ -> [_ _ _ _ _ _ _ _ _ _ _ _ _ _]
      dyn-events: _ -> [_ _ _ _ _ _ _ _ _ _ _ _ _ _]
      timeout: _ -> [_ _ _ _ _ _ _ _ _ _ _ _ _ _]
      tunnel: w583 -> [_ _ _ _ _ _ _ _ w597 _ w604 _ _ _]
      tunnel: w582 -> [_ _ _ _ _ _ _ _ _ _ w603 _ _ _]
      tunnel: w581 -> [_ _ _ _ _ _ _ _ _ _ _ w624 _ _]
      tunnel: w580 -> [_ _ _ _ _ _ _ _ _ _ _ _ w630 _]
      event Timeout {
        n315 = event-data() -> ()  [unwired: 1 in, 3 out]
      }
      event "流程操作": Value Change {
        n316 = event-data() -> ()  [unwired: 1 in, 6 out]
        n317 = global read "总磷总氮断电保存全局变量.vi" "简易流程路径"() -> (w585:path)
        n318 = global read "总磷总氮断电保存全局变量.vi" "流程路径"() -> (w586:path)
        n319 = call "流程批量写入.vi"("简易流程路径"=w585, "添加的路径"=w586) -> ()  [unwired: 10 in]
      }
      event "温度曲线": Value Change {
        n320 = event-data() -> ()  [unwired: 1 in, 6 out]
        n321 = call "温度曲线显示.vi"() -> ()  [unwired: 12 in]
      }
      event "试剂余量": Value Change {
        n322 = event-data() -> ()  [unwired: 1 in, 6 out]
        n323 = call "试剂余量显示UI.vi"() -> ()  [unwired: 12 in]
      }
      event "灯值调整": Value Change {
        n324 = event-data() -> ()  [unwired: 1 in, 6 out]
        n325 = call "灯值调整对话框.vi"() -> ()  [unwired: 12 in]
      }
      event "布尔": Value Change {
        n326 = event-data() -> ("NewVal"=w587:bool)  [unwired: 1 in, 5 out]
        n327 = case shown="假" w587 {
          frame False {
            n328 = global write "VAR总磷总氮全局变量.vi" "权限等级"(enum16{"一级权限", "二级权限", "三级权限", "超级权限"}."一级权限" ("权限等级")) -> ()
          }
          frame True {
            n329 = global read "VAR总磷总氮全局变量.vi" "权限密码"() -> (w591:u32[])
            n330 = global read "VAR总磷总氮全局变量.vi" "权限等级"() -> (w589:enum16{"一级权限", "二级权限", "三级权限", "超级权限"})
            n331 = call "密码权限设置.vi"("权限输入"=w589, "权限密码"=w591) -> ("权限输出"=w590:enum16{"一级权限", "二级权限", "三级权限", "超级权限"})  [unwired: 9 in]
            n332 = global write "VAR总磷总氮全局变量.vi" "权限等级"(w590) -> ()
          }
        }
      }
      event "权限等级": Mouse Down {
        n333 = event-data() -> ()  [unwired: 1 in, 8 out]
        n334 = global read "VAR总磷总氮全局变量.vi" "权限密码"() -> (w594:u32[])
        n335 = global read "VAR总磷总氮全局变量.vi" "权限等级"() -> (w592:enum16{"一级权限", "二级权限", "三级权限", "超级权限"})
        n336 = call "密码权限设置.vi"("权限输入"=w592, "权限密码"=w594) -> ("权限输出"=w593:enum16{"一级权限", "二级权限", "三级权限", "超级权限"})  [unwired: 9 in]
        n337 = global write "VAR总磷总氮全局变量.vi" "权限等级"(w593) -> ()
      }
      event "外设固件": Value Change {
        n338 = event-data() -> ()  [unwired: 1 in, 6 out]
        n339 = call "流程固件设置对话框.vi"() -> ()  [unwired: 12 in]
      }
      event "手动启动": Value Change {
        n340 = event-data() -> ()  [unwired: 1 in, 6 out]
        n341 = call "总磷总氮启动参数对话框.vi"() -> ("确认"=w595:bool, "元素"=w596:cluster{"命令":string, "data":variant})  [unwired: 10 in]
        n342 = case shown="真" w595 {
          tunnel: w597 -> [_ w600]
          tunnel: w596 -> [_ w599]
          frame False {
          }
          frame True {
            n343 = Flush Queue(queue=w600) -> (queue out=w598:refnum<queue>)  [unwired: 1 in, 2 out]
            n344 = Enqueue Element(queue=w598, element=w599) -> ()  [unwired: 2 in, 3 out]
          }
        }
      }
      event "调试": Value Change {
        n345 = event-data() -> ()  [unwired: 1 in, 6 out]
        n346 = call "简易流程调试界面.vi"() -> ()  [unwired: 12 in]
      }
      event "停止": Value Change {
        n347 = event-data() -> ()  [unwired: 1 in, 6 out]
        n348 = Two Button Dialog(message="确认停止？" ("消息")) -> (T button?=w601:bool)  [unwired: 2 in]
        n349 = case shown="真" w601 {
          tunnel: w604 -> [_ w620]
          tunnel: w603 -> [_ w619]
          frame False {
          }
          frame True {
            n350 = Send Notification(notification=TRUE ("通知"), notifier=w619) -> ()  [unwired: 1 in, 2 out]
            n351 = global read "VAR总磷总氮全局变量.vi" "状态告警区"() -> (w614:T5)
            n352 = global read "VAR总磷总氮全局变量.vi" "状态告警区"() -> (w606:T5)
            n353 = Unbundle By Name(w614) -> ("id"=w613:u16)
            n354 = Unbundle By Name(w606) -> ("id"=w605:u16)
            n355 = Bundle By Name(cluster=T18 {"站号"=1, "量程切换"=enum."AUTO", "控制命令"=enum."停止测试", "模式设置"=enum."待机", "测量间隔"=0} ("参数"), "站号"=w613) -> (w615:T18)
            n356 = call "id参数转换.vi"("id"=w605) -> ("table输出"=w607:string)  [unwired: 9 in, 1 out]
            n357 = call "总磷总氮启动命令.vi"("参数"=w615) -> ("启动命令"=w616:cluster{"命令":string, "data":variant})  [unwired: 10 in]
            n358 = Get Date/Time In Seconds() -> (seconds since 1Jan1904=w610:timestamp)
            n359 = Bundle By Name(cluster=T17 {"时间"=timestamp(0 s since 1904-01-01), "参数"="", "日志信息"="", "流程参数"=""} ("data in"), "时间"=w610, "参数"=w607, "日志信息"="手动停止") -> (w611:T17)
            n360 = Enqueue Element(queue=w620, element=w616) -> (error out=w608:errorcluster)  [unwired: 2 in, 2 out]
            n361 = call "总磷总氮操作日志.vi"("错误输入（无错误）"=w608, "data in"=w611) -> ()  [unwired: 9 in, 1 out]
          }
        }
      }
      event "参数设置", "参数查询": Value Change {
        n362 = event-data() -> ()  [unwired: 1 in, 6 out]
        n363 = invoke on="子面板" class="SubPnl" method="Remove VI"() -> (error out=w625:errorcluster)  [unwired: 3 in, 2 out]
        n364 = property on="仪器校准" class="Bool"("Visible"=TRUE ("可见")) -> ()  [unwired: 2 in, 2 out]
        n365 = property on="参数查询" class="Bool"("Visible"=FALSE ("可见")) -> ()  [unwired: 2 in, 2 out]
        n366 = property on="窗格" class="Pane"("Origin"=T7 {"Horizontal"=0, "Vertical"=640} ("原点")) -> ()  [unwired: 2 in, 2 out]
        n367 = invoke on="子面板" class="SubPnl" method="Insert VI"(error in=w625, "VI Ref"=w624) -> ()  [unwired: 2 in, 4 out]
        n368 = global write "VAR总磷总氮全局变量.vi" "页面"(enum16{"主页", "参数页", "校准页"}."参数页" ("页面")) -> ()
      }
      event "仪器校准": Value Change {
        n369 = event-data() -> ()  [unwired: 1 in, 6 out]
        n370 = invoke on="子面板" class="SubPnl" method="Remove VI"() -> (error out=w631:errorcluster)  [unwired: 3 in, 2 out]
        n371 = property on="仪器校准" class="Bool"("Visible"=FALSE ("可见")) -> ()  [unwired: 2 in, 2 out]
        n372 = property on="参数查询" class="Bool"("Visible"=TRUE ("可见")) -> ()  [unwired: 2 in, 2 out]
        n373 = global write "VAR总磷总氮全局变量.vi" "页面"(enum16{"主页", "参数页", "校准页"}."校准页" ("页面")) -> ()
        n374 = invoke on="子面板" class="SubPnl" method="Insert VI"(error in=w631, "VI Ref"=w630) -> ()  [unwired: 2 in, 4 out]
      }
      event "返回": Value Change {
        n375 = event-data() -> ()  [unwired: 1 in, 6 out]
        n376 = global write "VAR总磷总氮全局变量.vi" "页面"(enum16{"主页", "参数页", "校准页"}."主页" ("页面")) -> ()
        n377 = property on="窗格" class="Pane"("Origin"=T7 {"Horizontal"=0, "Vertical"=0} ("原点")) -> ()  [unwired: 2 in, 2 out]
      }
    }
  }
  n378 = while {
    tunnel: w20 -> [w645]
    stop <- FALSE stop-if-true
    n379 = Wait (ms)(milliseconds to wait=u32 1000 ("等待时间（毫秒）")) -> ()  [unwired: 1 out]
    n380 = global read "总磷总氮断电保存全局变量.vi" "MB通信方式选择"() -> (w643:enum16{"串口", "TCP"})
    n381 = global read "VAR总磷总氮全局变量.vi" "升级固件关闭心跳包"() -> (w637:bool)
    n382 = global read "VAR总磷总氮全局变量.vi" "MB session in"() -> (w641:refnum<class "MB_Master.lvclass">)
    n383 = case shown="\"串口\", 默认" w643 {
      tunnel: [w648 w649] -> w642
      frame "串口", Default {
        n384 = global read "总磷总氮断电保存全局变量.vi" "VISA Resource"() -> (w648:refnum<visa-resource-name>)
      }
      frame "TCP" {
        n385 = global read "总磷总氮断电保存全局变量.vi" "IP"() -> (w649:string)
      }
    }
    "字符串 2" <- w642
    n386 = property class="MB_Master"(reference=w641) -> ("Properties:Session Valid"=w639:bool)  [unwired: 1 in, 2 out]
    n387 = Not(x=w637) -> (.not. x?=w636:bool)
    n388 = Get Queue Status(queue=w645) -> (queue out=w644:refnum<queue>, # elements in queue=w640:i32)  [unwired: 2 in, 6 out]
    n389 = Equal To 0?(x=w640) -> (x = 0?=w634:bool)
    n390 = Compound Arithmetic op=AND ("复合运算")(w639, w636) -> (w638:bool)
    n391 = global write "VAR总磷总氮全局变量.vi" "心跳包打开状态"(w638) -> ()
    n392 = And(x=w634, y=w638) -> (x .and. y?=w635:bool)
    n393 = case shown="真" w635 {
      tunnel: w644 -> [_ w668]
      frame False {
      }
      frame True {
        n394 = global read "VAR总磷总氮全局变量.vi" "MB session in"() -> (w656:refnum<class "MB_Master.lvclass">)
        n395 = property class="MB_Master"(reference=w656) -> ("Properties:Session Valid"=w654:bool)  [unwired: 1 in, 2 out]
        n396 = global read "VAR总磷总氮全局变量.vi" "通讯状态"() -> (w657:bool)
        n397 = case shown="真" w654 {
          tunnel: [_ w670] -> w653
          frame False {
          }
          frame True {
            n398 = global read "VAR总磷总氮全局变量.vi" "MB session in"() -> (w669:refnum<class "MB_Master.lvclass">)
            n399 = call "版本号读取.vi"("MB session in"=w669) -> ("error out"=w670:errorcluster, "固件版本号"=w671:string)  [unwired: 8 in, 1 out]
            "固件版本号" <- w671
            n400 = global write "VAR总磷总氮全局变量.vi" "固件版本号"(w671) -> ()
          }
        }
        n401 = And(x=w654, y=w657) -> (x .and. y?=w655:bool)
        n402 = case shown="真" w655 {
          tunnel: [_ w672] -> w652
          tunnel: w653 -> [_ w673]
          frame False {
          }
          frame True {
            n403 = global read "VAR总磷总氮全局变量.vi" "MB session in"() -> (w675:refnum<class "MB_Master.lvclass">)
            n404 = call "序列号读取.vi"("Error in"=w673, "MB session in"=w675) -> ("error out"=w672:errorcluster, "序列号"=w674:string)  [unwired: 7 in, 1 out]
            n405 = global write "VAR总磷总氮全局变量.vi" "序列号"(w674) -> ()
          }
        }
        n406 = global read "model config var.vi" "启动队列名称"() -> (w659:cluster{"String":string, "Value":u16}[])
        n407 = for {
          tunnel: [w686] -> w660 mode=indexing
          tunnel: w659 -> [w687] mode=indexing
          tunnel: w652 -> [_]
          n408 = Unbundle By Name(w687) -> ("Value"=w686:u16)
        }
        n409 = for {
          shift-right: [w676] -> w662
          shift-left: w668 -> [w682]
          tunnel: w660 -> [w677] mode=indexing
          n410 = Bundle By Name(cluster=cluster{"命令":string, "data":variant} {"命令"="", "data"=variant} ("元素"), "命令"="读状态告警区", "data"=w677) -> (w684:cluster{"命令":string, "data":variant})
          n411 = Bundle By Name(cluster=cluster{"命令":string, "data":variant} {"命令"="", "data"=variant} ("元素"), "命令"="读测量数据区", "data"=w677) -> (w679:cluster{"命令":string, "data":variant})
          n412 = Enqueue Element(queue=w682, element=w684) -> (queue out=w678:refnum<queue>)  [unwired: 2 in, 2 out]
          n413 = Enqueue Element At Opposite End(queue=w678, element=w679) -> (queue out=w676:refnum<queue>)  [unwired: 2 in, 2 out]
        }
        n414 = global read "VAR总磷总氮全局变量.vi" "状态告警区"() -> (w661:T5)
        n415 = Unbundle By Name(w661) -> ("系统时间"=w650:timestamp)
        n416 = Get Date/Time In Seconds() -> (seconds since 1Jan1904=w667:timestamp)
        n417 = Subtract(x=w667, y=w650) -> (x-y=w666:dbl)
        n418 = Absolute Value(x=w666) -> (abs(x)=w665:dbl)
        n419 = global read "VAR总磷总氮全局变量.vi" "通讯状态"() -> (w651:bool)
        n420 = Greater Or Equal?(x=w665, y=30.0) -> (x >= y?=w663:bool)
        n421 = Compound Arithmetic op=AND ("复合运算")(w663, w651) -> (w658:bool)
        n422 = case shown="真" w658 {
          tunnel: w662 -> [_ w689]
          frame False {
          }
          frame True {
            n423 = call "总磷总氮启动命令.vi"("参数"=T18 {"站号"=3, "量程切换"=enum."AUTO", "控制命令"=enum."校时", "模式设置"=enum."待机", "测量间隔"=0}) -> ("启动命令"=w688:cluster{"命令":string, "data":variant})  [unwired: 10 in]
            n424 = Enqueue Element(queue=w689, element=w688) -> ()  [unwired: 2 in, 3 out]
          }
        }
      }
    }
  }
